vi "Get SubPicture Coordinates.vi"(11 "24-bit pixmap":u32[][](array[numeric])) -> (0 "b-a":i32, 2 "b":i32, 3 "a":i32)   [LabVIEW 2020, in "lv_icon.lvlib"]
doc: "Get multiple sub-picture coordinates."
uses:
  lv_icon.lvlib
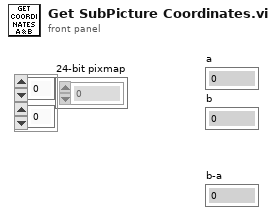
[diagram p1: front panel]
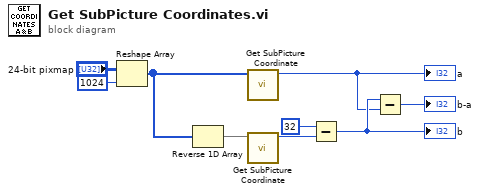
[diagram p0: block diagram]
diagram:
  n1 = Reshape Array("24-bit pixmap", 1024 ("dimension size")) -> (w8:u32[])
  n2 = Reverse 1D Array(array=w8) -> (reversed array=w9:u32[])
  n3 = call "Get SubPicture Coordinate.vi"("Image in"=w8) -> ("quotient"=w2:i32)  [unwired: 10 out]
  "a" <- w2
  n4 = call "Get SubPicture Coordinate.vi"("Image in"=w9) -> ("quotient"=w4:i32)  [unwired: 10 out]
  n5 = Subtract(x=32, y=w4) -> (x-y=w3:i32)
  "b" <- w3
  n6 = Subtract(x=w3, y=w2) -> (x-y=→"b-a":i32)
